vi "Get Manual Observer.vi"(8 "error in (no error)":errorcluster, 11 "Vessel in":refnum<class "Vessel.lvclass">) -> (0 "error out":errorcluster, 2 "Active Observer":refnum<class "Observer.lvclass">, 3 "Vessel out":refnum<class "Vessel.lvclass">)   [LabVIEW 2014, in "Vessel.lvclass"]
uses:
  Vessel.lvclass
  Observer/Observer.lvclass
  Supervisor/Supervisor.lvclass
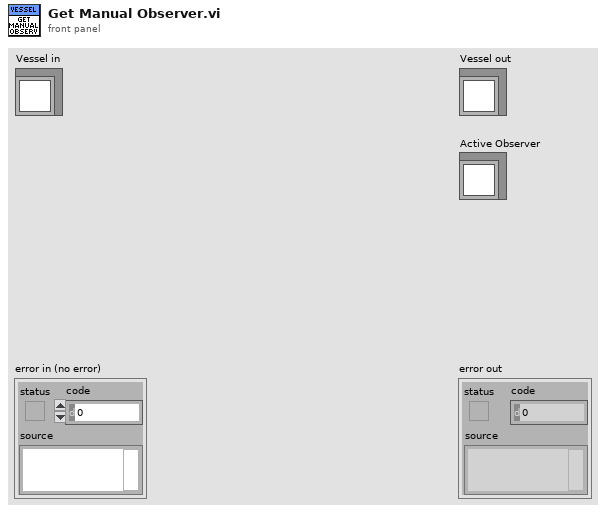
[diagram p1: front panel]
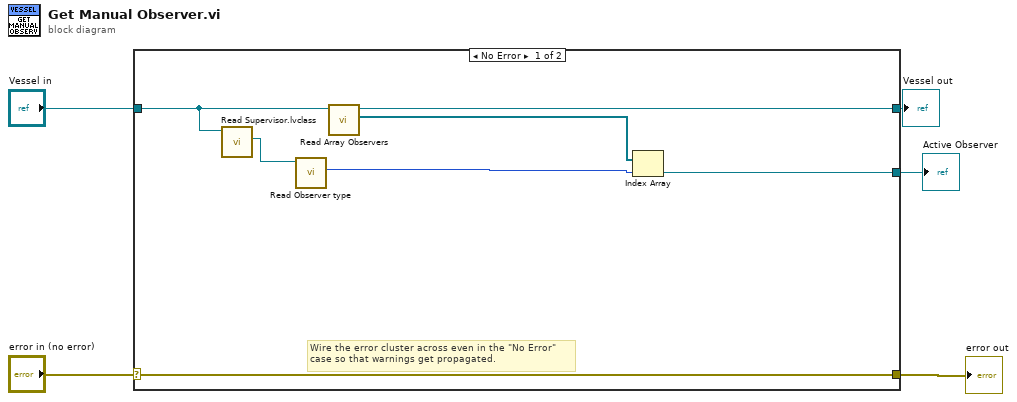
[diagram p0: block diagram]
diagram:
  n1 = case shown="No Error" "error in (no error)" {
    selector: "error in (no error)" -> [w12 w14]
    tunnel: [w12 w14] -> w4
    tunnel: [w10 w13] -> w2
    tunnel: "Vessel in" -> [w11 w13]
    tunnel: [w8 _] -> w1
    frame No Error {
      # "Wire the error cluster across even in the \"No Error\"\ncase so that warnings get propagated."
      n2 = call "Read Supervisor.lvclass.vi"("Vessel in"=w11) -> ("Supervisor.lvclass"=w7:refnum<class "Supervisor.lvclass">)  [unwired: 8 in, 2 out]
      n3 = call-dynamic "Read Observer type.vi"("Supervisor in"=w7) -> ("Observer type"=w6:i16)  [unwired: 8 in, 2 out]
      n4 = call-dynamic "Read Array Observers.vi"("Vessel in"=w11) -> ("Array Observers"=w9:refnum<class "Observer.lvclass">[], "Vessel out"=w10:refnum<class "Vessel.lvclass">)  [unwired: 8 in, 1 out]
      n5 = Index Array(array=w9, index=w6) -> (element=w8:refnum<class "Observer.lvclass">)
    }
    frame Error {
    }
  }
  "error out" <- w4
  "Vessel out" <- w2
  "Active Observer" <- w1
